vi "Table_InitializeListboxCellColor.vi"(8 "error in (no error)":errorcluster, 10 "Array Size":i32, 11 "Listbox Ref":refnum<vi>) -> (0 "error out":errorcluster, 3 "Listbox Ref Out":refnum<vi>)   [LabVIEW 2012, in "TableSupportLib.lvlib"]
uses:
  <vilib>/Utility/miscctls.llb/LVRowAndColumnTypeDef.ctl
  TableSupportLib.lvlib
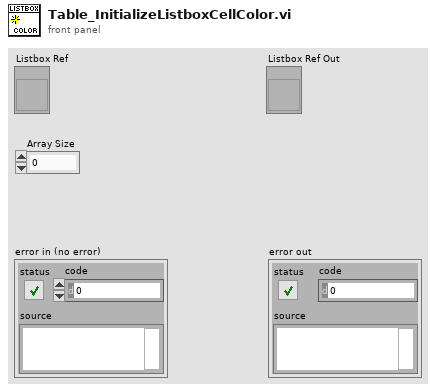
[diagram p1: front panel]
types:
  T1 = typedef "LVRowAndColumnTypeDef.ctl" = cluster{"Row":i32, "Column":i32}
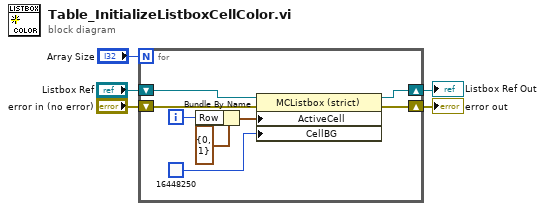
[diagram p0: block diagram]
diagram:
  n1 = for {
    N: "Array Size" -> [_]
    shift-right: [w7] -> w3
    shift-left: "error in (no error)" -> [w9]
    shift-right: [w8] -> w2
    shift-left: "Listbox Ref" -> [w10]
    i -> [w6]
    n2 = Bundle By Name(cluster=T1 {"Row"=0, "Column"=1} ("Active Cell:Active Cell"), "Row"=w6) -> (w12:T1)
    n3 = property on="Property Node" class="MCListbox (strict)"(reference=w10, error in=w9, "ActiveCell"=w12, "CellBG"=u32 16448250) -> (reference out=w8:refnum<vi>, error out=w7:errorcluster)
  }
  "error out" <- w3
  "Listbox Ref Out" <- w2
